vi "Trololololololololololololololololololol.vi"() -> (0 "Message":string)   [LabVIEW 2015]
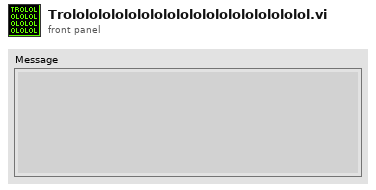
[diagram p1: front panel]
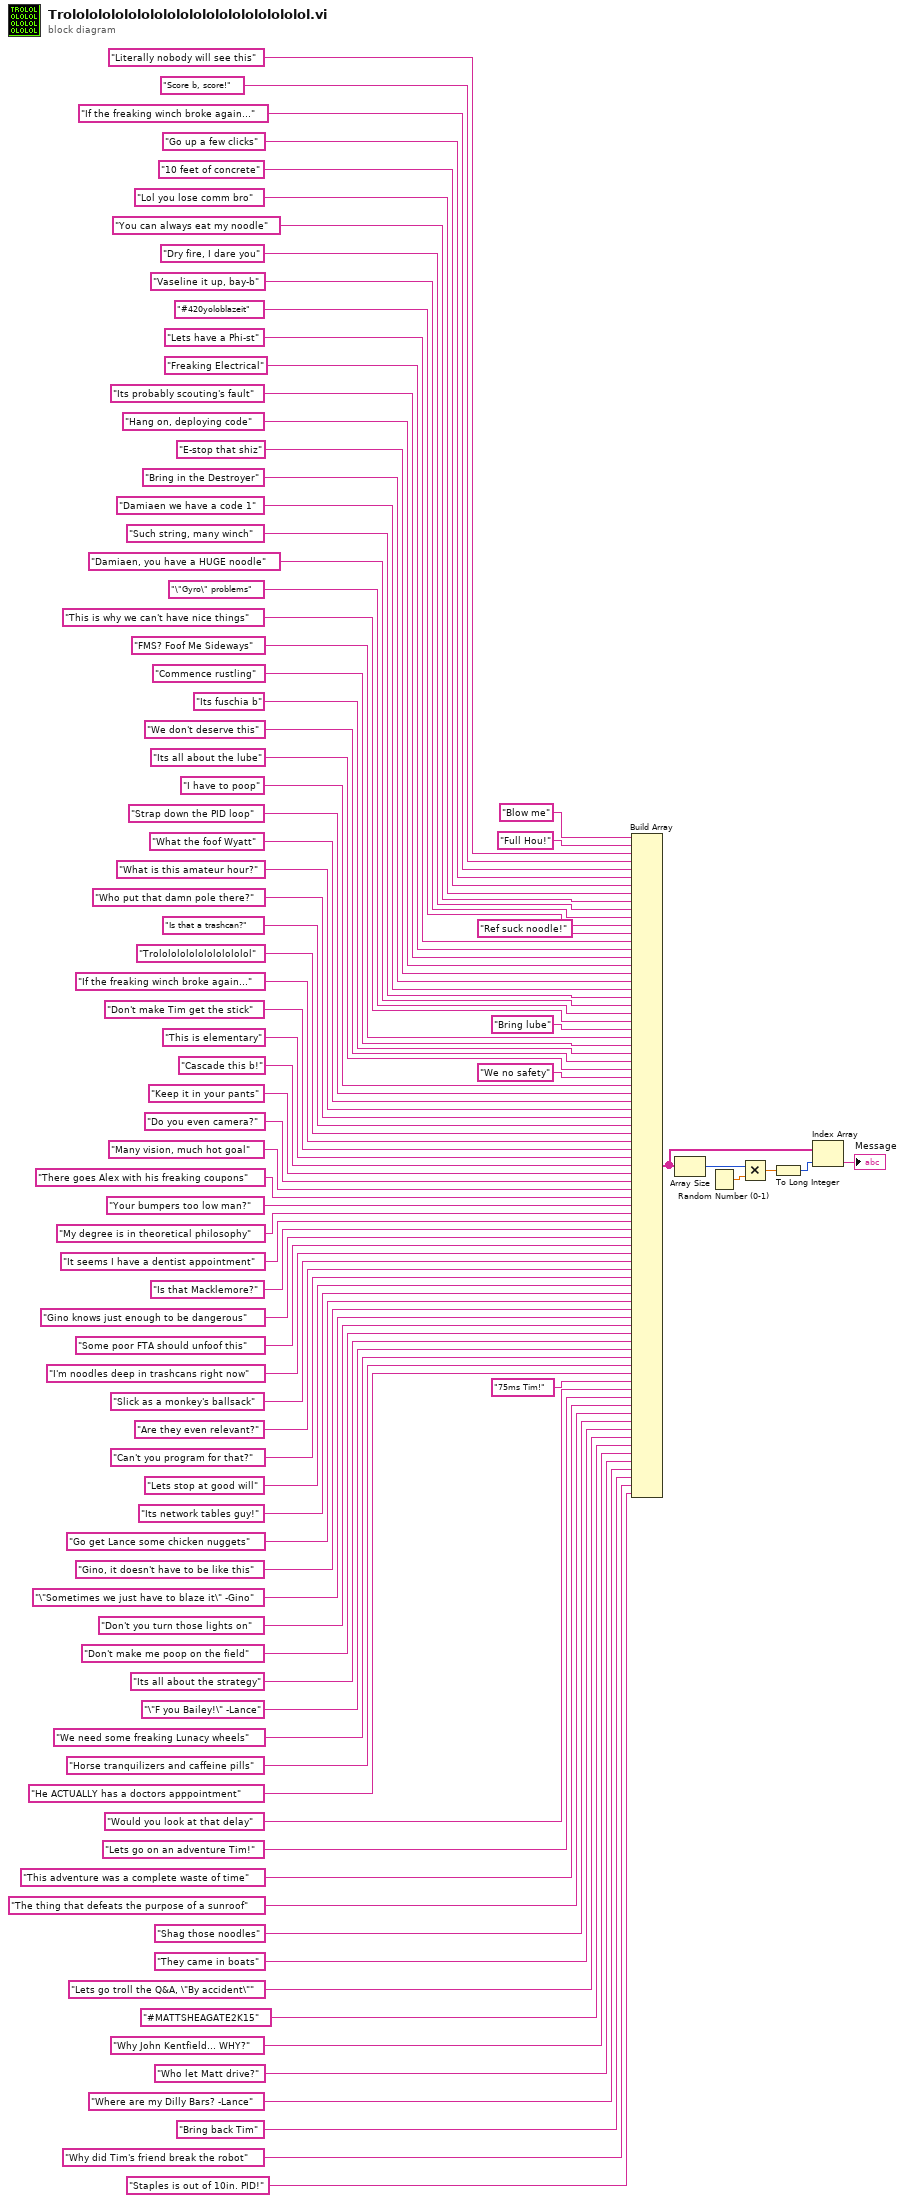
[diagram p0: block diagram]
diagram:
  n1 = Build Array("Blow me" ("element"), "Full Hou!", "Literally nobody will see this" ("element"), "Score b, score!", "If the freaking winch broke again...", "Go up a few clicks", "10 feet of concrete", "Lol you lose comm bro", "You can always eat my noodle", "Dry fire, I dare you", "Vaseline it up, bay-b", "#420yoloblazeit", "Ref suck noodle!", "Lets have a Phi-st", "Freaking Electrical", "Its probably scouting's fault", "Hang on, deploying code", "E-stop that shiz", "Bring in the Destroyer", "Damiaen we have a code 1", "Such string, many winch" ("element"), "Damiaen, you have a HUGE noodle", "\"Gyro\" problems" ("element"), "This is why we can't have nice things" ("element"), "Bring lube" ("element"), "FMS? Foof Me Sideways" ("element"), "Commence rustling" ("element"), "Its fuschia b" ("element"), "We don't deserve this" ("element"), "Its all about the lube" ("element"), "We no safety" ("element"), "I have to poop" ("element"), "Strap down the PID loop" ("element"), "What the foof Wyatt" ("element"), "What is this amateur hour?" ("element"), "Who put that damn pole there?" ("element"), "Is that a trashcan?" ("element"), "Trololololololololololol" ("element"), "If the freaking winch broke again..." ("element"), "Don't make Tim get the stick" ("element"), "This is elementary" ("element"), "Cascade this b!" ("element"), "Keep it in your pants" ("element"), "Do you even camera?" ("element"), "Many vision, much hot goal" ("element"), "There goes Alex with his freaking coupons" ("element"), "Your bumpers too low man?" ("element"), "My degree is in theoretical philosophy" ("element"), "It seems I have a dentist appointment" ("element"), "Is that Macklemore?" ("element"), "Gino knows just enough to be dangerous" ("element"), "Some poor FTA should unfoof this" ("element"), "I'm noodles deep in trashcans right now" ("element"), "Slick as a monkey's ballsack" ("element"), "Are they even relevant?" ("element"), "Can't you program for that?" ("element"), "Lets stop at good will" ("element"), "Its network tables guy!" ("element"), "Go get Lance some chicken nuggets" ("element"), "Gino, it doesn't have to be like this" ("element"), "\"Sometimes we just have to blaze it\" -Gino" ("element"), "Don't you turn those lights on" ("element"), "Don't make me poop on the field" ("element"), "Its all about the strategy" ("element"), "\"F you Bailey!\" -Lance" ("element"), "We need some freaking Lunacy wheels" ("element"), "Horse tranquilizers and caffeine pills" ("element"), "He ACTUALLY has a doctors apppointment" ("element"), "75ms Tim!" ("element"), "Would you look at that delay" ("element"), "Lets go on an adventure Tim!" ("element"), "This adventure was a complete waste of time" ("element"), "The thing that defeats the purpose of a sunroof" ("element"), "Shag those noodles" ("element"), "They came in boats" ("element"), "Lets go troll the Q&A, \"By accident\"", "#MATTSHEAGATE2K15", "Why John Kentfield... WHY?", "Who let Matt drive?", "Where are my Dilly Bars? -Lance", "Bring back Tim", "Why did Tim's friend break the robot", "Staples is out of 10in. PID!") -> (w14:string[])
  n2 = Array Size(array=w14) -> (size(s)=w5:i32)
  n3 = Random Number (0-1)() -> (number: 0 to 1=w4:dbl)
  n4 = Multiply(x=w5, y=w4) -> (x*y=w3:dbl)
  n5 = To Long Integer(number=w3) -> (32bit integer=w2:i32)
  n6 = Index Array(array=w14, index=w2) -> (element=→"Message":string)
